vi "Pad Analyzer Region.vi"(4 "Analyzer Region":T2) -> (1 "Analyzer Region out":T1)   [LabVIEW 2018]
panel:
  in  "@dummy control@":i8
  in  "@dummy control@":i8
  in  "@dummy control@":i8
  in  "@dummy control@":i8
  in  "@dummy control@":i8
  in  "@dummy control@":i8
  in  "@dummy control@":i8
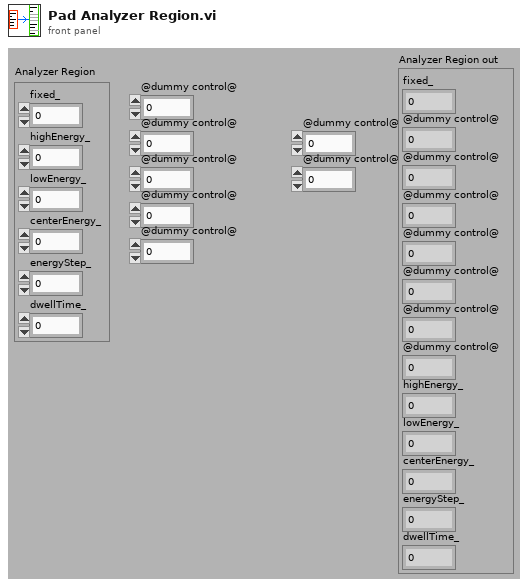
[diagram p1: front panel]
types:
  T1 = cluster{"fixed_":u8, "@dummy control@":i8, "@dummy control@":i8, "@dummy control@":i8, "@dummy control@":i8, "@dummy control@":i8, "@dummy control@":i8, "@dummy control@":i8, "highEnergy_":dbl, "lowEnergy_":dbl, "centerEnergy_":dbl, "energyStep_":dbl, "dwellTime_":i32}
  T2 = cluster{"fixed_":u8, "highEnergy_":dbl, "lowEnergy_":dbl, "centerEnergy_":dbl, "energyStep_":dbl, "dwellTime_":i32}
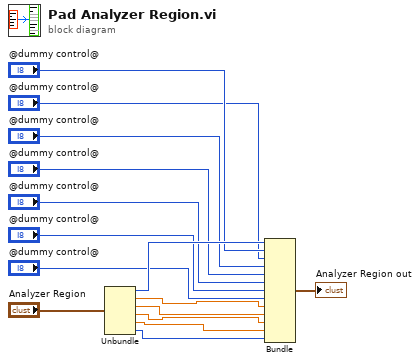
[diagram p0: block diagram]
diagram:
  n1 = Unbundle("Analyzer Region") -> ("fixed_"=w14:u8, "highEnergy_"=w13:dbl, "lowEnergy_"=w12:dbl, "centerEnergy_"=w11:dbl, "energyStep_"=w10:dbl, "dwellTime_"=w9:i32)
  n2 = Bundle("fixed_"=w14, "@dummy control@"="@dummy control@", "@dummy control@"="@dummy control@", "@dummy control@"="@dummy control@", "@dummy control@"="@dummy control@", "@dummy control@"="@dummy control@", "@dummy control@"="@dummy control@", "@dummy control@"="@dummy control@", "highEnergy_"=w13, "lowEnergy_"=w12, "centerEnergy_"=w11, "energyStep_"=w10, "dwellTime_"=w9) -> (→"Analyzer Region out":T1)  [unwired: 1 in]
